vi "Extract URI Components.vi"(8 "error in":errorcluster, 11 "URI":string="https://tools.ietf.org:80/html/rfc3986?query=test&query2=test2#appendix-A") -> (0 "error out":errorcluster, 3 "URI Components":T1)   [LabVIEW 2013, in "openURI.lvlib"]
uses:
  openURI.lvlib
  URI Components -- cluster.ctl
  <vilib>/regexp/Match Regular Expression.xnode
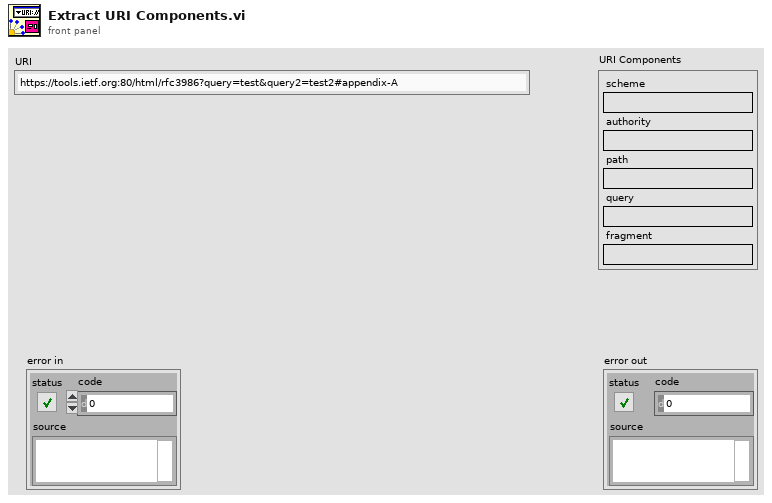
[diagram p1: front panel]
types:
  T1 = typedef "openURI.lvlib/URI Components -- cluster.ctl" = cluster{"scheme":string, "authority":string, "path":string, "query":string, "fragment":string}
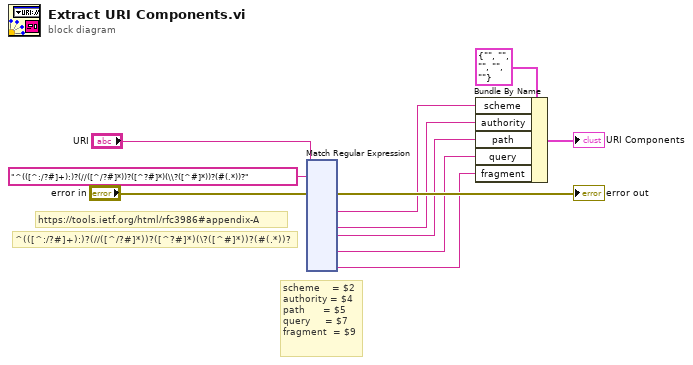
[diagram p0: block diagram]
diagram:
  # "https://tools.ietf.org/html/rfc3986#appendix-A"
  # "scheme    = $2\nauthority = $4\npath      = $5\nquery     = $7\nfragment  = $9"
  # "^(([^:/?#]+):)?(//([^/?#]*))?([^?#]*)(\\?([^#]*))?(#(.*))?"
  n1 = xnode "Match Regular Expression"("input string"="URI", "regular expression"="^(([^:/?#]+):)?(//([^/?#]*))?([^?#]*)(\\?([^#]*))?(#(.*))?", "error in"="error in") -> ("error out"=→"error out":errorcluster, "submatch 2"=w6:string, "submatch 4"=w5:string, "submatch 5"=w4:string, "submatch 7"=w3:string, "submatch 9"=w2:string)  [unwired: 3 in, 8 out]
  n2 = Bundle By Name(cluster=T1 {"scheme"="", "authority"="", "path"="", "query"="", "fragment"=""} ("URI Components"), "scheme"=w6, "authority"=w5, "path"=w4, "query"=w3, "fragment"=w2) -> (→"URI Components":T1)
